vi "Event Handle Loop_Startup.vi"(8 "error in (no error)":errorcluster, 11 "QTab Class in":refnum<class "QTab Class.lvclass">) -> (0 "error out":errorcluster, 3 "QTab Class out":refnum<class "QTab Class.lvclass">)   [LabVIEW 2020, in "QTab.lvlib" / "QTab Class.lvclass"]
uses:
  QTab Class.lvclass
  QTab Class.lvclass/QTab Class.ctl
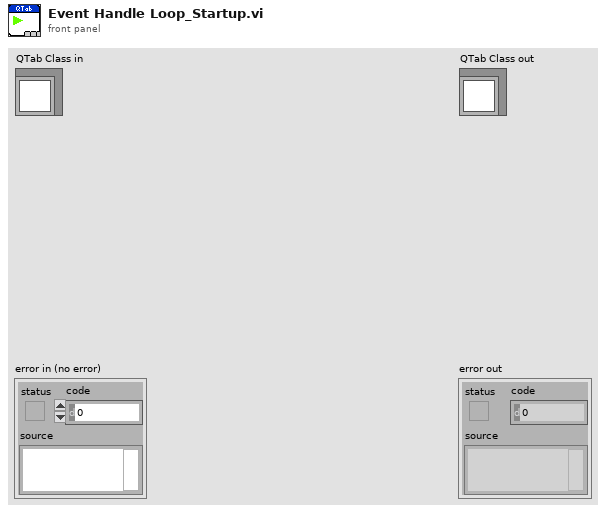
[diagram p1: front panel]
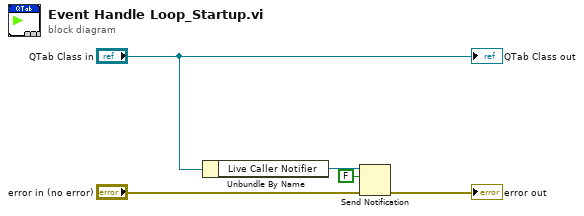
[diagram p0: block diagram]
diagram:
  n1 = Unbundle By Name("QTab Class in") -> ("Live Caller Notifier"=w3:refnum<notifier>)
  n2 = Send Notification(notification=FALSE, notifier=w3, error in (no error)="error in (no error)") -> (error out=→"error out":errorcluster)  [unwired: 1 out]
  "QTab Class out" <- "QTab Class in"
